vi "Configure Carrier (List Property).vi"(0 "VISA resource name":refnum<visa-resource-name>, 1 "Enable Carrier Coupling List":bool[](array[boolean])=[TRUE, TRUE], 2 "Measurement Noise Bandwidth List":dbl[](array[numeric])=[2000000.0, 2000000.0] format="%#.6g", 5 "Device Mode (1: BTS)":i32(ring)=1 items=["BTS"=1, "MS"=2], 7 "Filter Alpha List":dbl[](array[numeric])=[0.22, 0.22] format="%#.6g", 9 "Carrier Spacing List":dbl[](array[numeric])=[5000000.0, 5000000.0] format="%#.6g", 11 "error in (no error)":errorcluster, 12 "Enable Carrier Power Present List":bool[](array[boolean])=[TRUE, TRUE], 13 "Method List":i32[](array[ring])=[0, 0] items=["IBW", "RRC"]) -> (4 "VISA resource name out":refnum<visa-resource-name>, 15 "error out":errorcluster)   [LabVIEW 2014, in "Agilent MXA Series.lvlib"]
doc: "Configures the Carriers List settings under ACP measurement type."
uses:
  Agilent MXA Series.lvlib
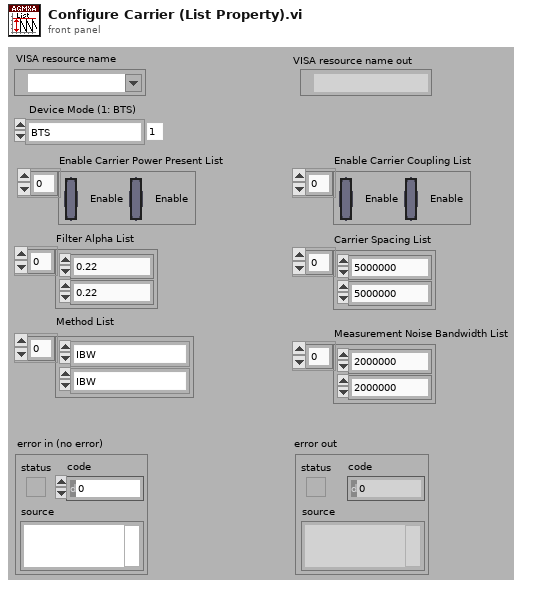
[diagram p1: front panel]
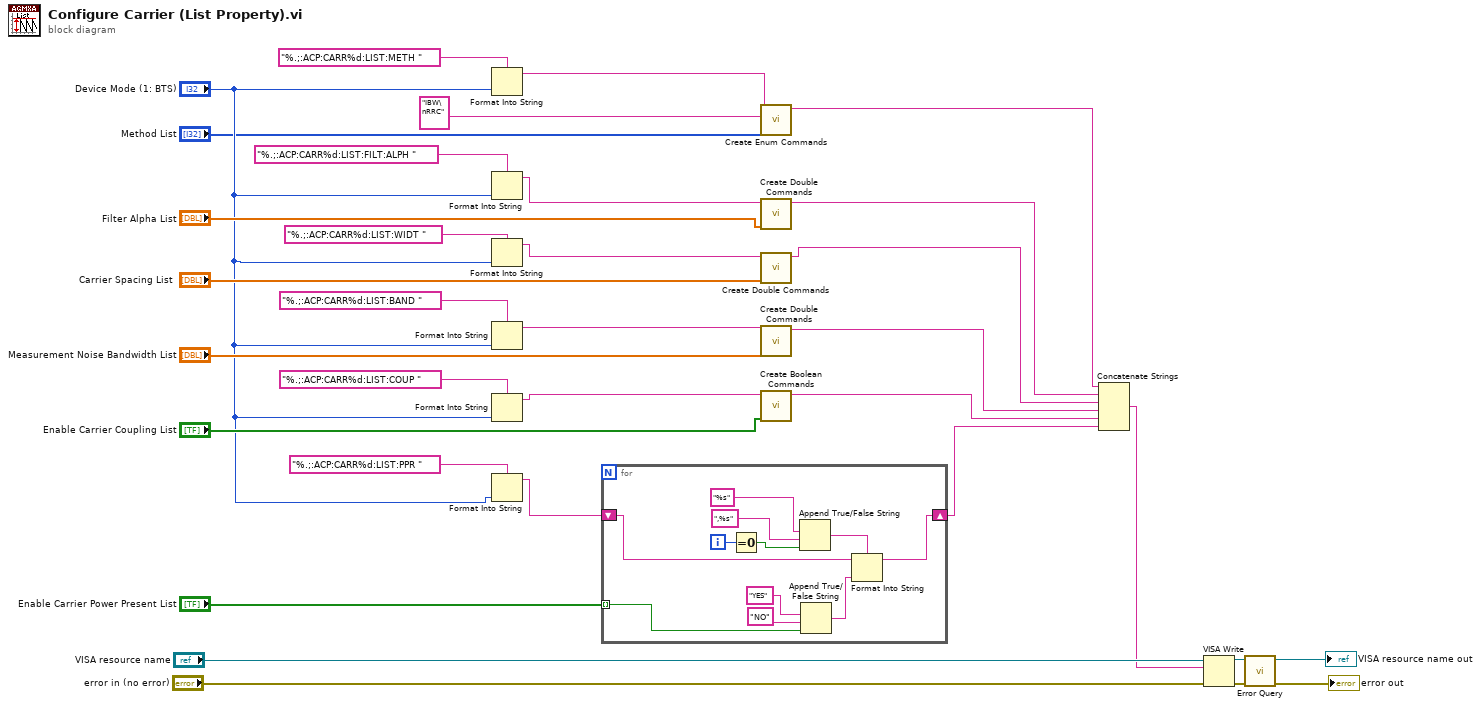
[diagram p0: block diagram]
diagram:
  n1 = Format Into String(format string="%.;:ACP:CARR%d:LIST:METH ", "Device Mode (1: BTS)") -> (resulting string=w5:string)  [unwired: 2 in, 1 out]
  n2 = Format Into String(format string="%.;:ACP:CARR%d:LIST:FILT:ALPH ", "Device Mode (1: BTS)") -> (resulting string=w30:string)  [unwired: 2 in, 1 out]
  n3 = Format Into String(format string="%.;:ACP:CARR%d:LIST:WIDT ", "Device Mode (1: BTS)") -> (resulting string=w28:string)  [unwired: 2 in, 1 out]
  n4 = Format Into String(format string="%.;:ACP:CARR%d:LIST:BAND ", "Device Mode (1: BTS)") -> (resulting string=w25:string)  [unwired: 2 in, 1 out]
  n5 = Format Into String(format string="%.;:ACP:CARR%d:LIST:COUP ", "Device Mode (1: BTS)") -> (resulting string=w22:string)  [unwired: 2 in, 1 out]
  n6 = Format Into String(format string="%.;:ACP:CARR%d:LIST:PPR ", "Device Mode (1: BTS)") -> (resulting string=w10:string)  [unwired: 2 in, 1 out]
  n7 = for {
    tunnel: "Enable Carrier Power Present List" -> [w36] mode=indexing
    shift-right: [w35] -> w8
    shift-left: w10 -> [w38]
    i -> [w40]
    n8 = Equal To 0?(x=w40) -> (x = 0?=w42:bool)
    n9 = Append True/False String(1:w42, 2:",%s" ("format string"), 3:"%s" ("format string")) -> (0:w39:string)  [unwired: 1 in]
    n10 = Append True/False String(1:w36, 2:"NO" ("multi-line string"), 3:"YES" ("true string")) -> (0:w37:string)  [unwired: 1 in]
    n11 = Format Into String(format string=w39, initial string=w38, w37) -> (resulting string=w35:string)  [unwired: 1 in, 1 out]
  }
  n12 = call "Create Enum Commands.vi"("Enum Values"="Method List", "Multi-line Text"="IBW\nRRC" ("multi-line string"), "Commands"=w5) -> ("Result"=w4:string)  [unwired: 8 in]
  n13 = call "Create Double Commands.vi"("Double Values"="Filter Alpha List", "Commands"=w30) -> ("Result"=w3:string)  [unwired: 9 in]
  n14 = call "Create Double Commands.vi"("Double Values"="Carrier Spacing List", "Commands"=w28) -> ("Result"=w2:string)  [unwired: 9 in]
  n15 = call "Create Double Commands.vi"("Double Values"="Measurement Noise Bandwidth List", "Commands"=w25) -> ("Result"=w18:string)  [unwired: 9 in]
  n16 = call "Create Boolean Commands.vi"("Boolean States"="Enable Carrier Coupling List", "Command"=w22) -> ("Result String"=w17:string)  [unwired: 9 in]
  n17 = Concatenate Strings(w4, w3, w2, w18, w17, w8) -> (w1:string)
  n18 = VISA Write(VISA resource name="VISA resource name", write buffer=w1, error in (no error)="error in (no error)") -> (VISA resource name out=w15:refnum<visa-resource-name>, error out=w16:errorcluster)  [unwired: 1 out]
  n19 = call "Error Query.vi"("error in (no error)"=w16, "VISA resource name"=w15) -> ("error out"=→"error out":errorcluster, "VISA resource name out"=→"VISA resource name out":refnum<visa-resource-name>)  [unwired: 6 in, 2 out]
